vi "Edgertronic-:get_current_settings copy.vi"(4 "GET Command":string="/get_current_settings", 5 "Setup":T1={"URL"="130.64.16.195", "remote port"=80, "mode (standard)"=enum."Standard"}) -> (0 "error out":errorcluster, 1 "Current Settings:":T2={"Connection Information:"="", "Requested Genlock "="20140911165611", "Min Frame Clocks "="20140911165611", "Is Seq Clk Freq "="20140911165611", "Pretrigger Frames "="20140911165611", "Duration "="20140911165611", "Overclock "="20140911165611", "Requested Horizontal "="20140911165611", "Frames "="20140911165611", "Requested Pretrigger "="20140911165611", "Words per Frame "="20140911165611", "Buffer End "="20140911165611", "Clocks per Frame  "="20140911165611", "Requested Duration "="20140911165611", "Pretrigger "="20140911165611", "Post-trigger Frames "="20140911165611", "Vertical "="20140911165611", "Requested Vertical "="20140911165611", "Reqested Frame Rate "="20140911165611", "Frame Rate "="20140911165611", "Horizontal "="20140911165611", "Clocks per Exposure "="20140911165611", "Digital Gain "="20140911165611", "Exposure "="20140911165611", "Genlock "="20140911165611", "Analog Gain "="20140911165611", "Subsample "="20140911165611", "Requested Exposure "="20140911165611", "Iso "="20140911165611", "Requested Overclock "="20140911165611", "Requested Subsample "="20140911165611", "Requested Iso"="20140911165611", "FPGA Temp"="20140911165611", "Posttrigger Duration"="20140911165611", "dacvrefadc"="20140911165611", "Is Temp"="20140911165611", "Pretrigger Duration"="20140911165611"}, 2 "Data Out from Camera":string="HTTP/1.0 200 OK\r\nContent-Type: text/html; charset=utf-8\r\nContent-Length: 313\r\nConnection: close\r\nDate: Tue, 16 Jun 2015 13:54:12 GMT\r\nServer: lighttpd/1.4.11 (edgertonic slow motion camera)\r\n\r\n{\"build_date\": \"20150112\", \"sw_build_date\": \"20140911165611\", \"fpga_initialized\": 1, \"hardware_revision\": 6, \"model_number\": 1, \"home_dir\": \"/home/root/ss-web\", \"ir_filter\": 1, \"mac_addr\": \"00:1B:C5:09:61:4D\", \"serial_console_enabled\": false, \"serial_number\": 333, \"fpga_version\": 70, \"hardware_configuration\": 1}")   [LabVIEW 2012]
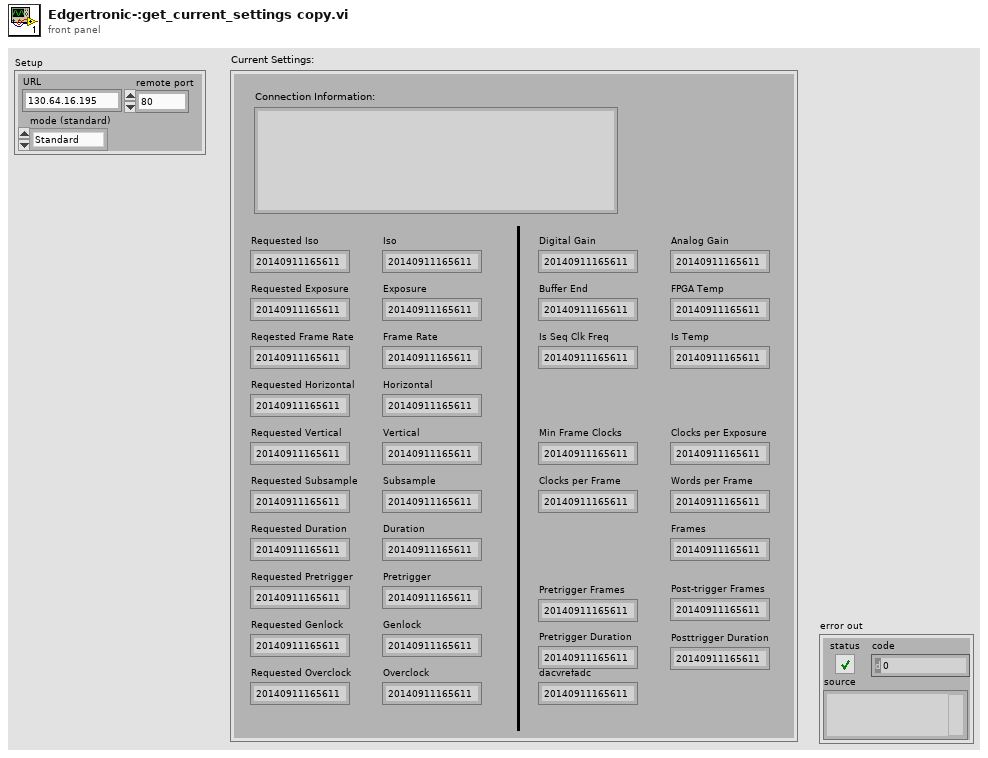
[diagram p1: front panel]
types:
  T1 = cluster{"URL":string, "remote port":u16, "mode (standard)":enum16{"Standard", "Buffered", "CRLF", "Immediate"}}
  T2 = cluster{"Connection Information:":string, "Requested Genlock ":string, "Min Frame Clocks ":string, "Is Seq Clk Freq ":string, "Pretrigger Frames ":string, "Duration ":string, "Overclock ":string, "Requested Horizontal ":string, "Frames ":string, "Requested Pretrigger ":string, "Words per Frame ":string, "Buffer End ":string, "Clocks per Frame  ":string, "Requested Duration ":string, "Pretrigger ":string, "Post-trigger Frames ":string, "Vertical ":string, "Requested Vertical ":string, "Reqested Frame Rate ":string, "Frame Rate ":string, "Horizontal ":string, "Clocks per Exposure ":string, "Digital Gain ":string, "Exposure ":string, "Genlock ":string, "Analog Gain ":string, "Subsample ":string, "Requested Exposure ":string, "Iso ":string, "Requested Overclock ":string, "Requested Subsample ":string, "Requested Iso":string, "FPGA Temp":string, "Posttrigger Duration":string, "dacvrefadc":string, "Is Temp":string, "Pretrigger Duration":string}
  T3 = cluster{"Parameter":string, "Parameter 2":string, "Parameter 3":string, "Parameter 4":string, "Parameter 5":string, "Parameter 6":string, "Parameter 7":string, "Parameter 8":string, "Parameter 9":string, "Parameter 10":string, "Parameter 11":string, "Parameter 12":string, "Parameter 13":string, "Parameter 14":string, "Parameter 15":string, "Parameter 16":string, "Parameter 17":string, "Parameter 18":string, "Parameter 19":string, "Parameter 20":string, "Parameter 21":string, "Parameter 22":string, "Parameter 23":string, "Parameter 24":string, "Parameter 25":string, "Parameter 26":string, "Parameter 27":string, "Parameter 28":string, "Parameter 29":string, "Parameter 30":string, "Parameter 31":string, "Parameter 32":string, "Parameter 33":string, "Parameter 34":string, "Parameter 35":string, "Parameter 36":string}
  T4 = cluster{"[0]":string, "[1]":string, "[2]":string, "[3]":string, "[4]":string, "[5]":string, "[6]":string, "[7]":string, "[8]":string, "[9]":string, "[10]":string, "[11]":string, "[12]":string, "[13]":string, "[14]":string, "[15]":string, "[16]":string, "[17]":string, "[18]":string, "[19]":string, "[20]":string, "[21]":string, "[22]":string, "[23]":string, "[24]":string, "[25]":string, "[26]":string, "[27]":string, "[28]":string, "[29]":string, "[30]":string, "[31]":string, "[32]":string, "[33]":string, "[34]":string, "[35]":string}
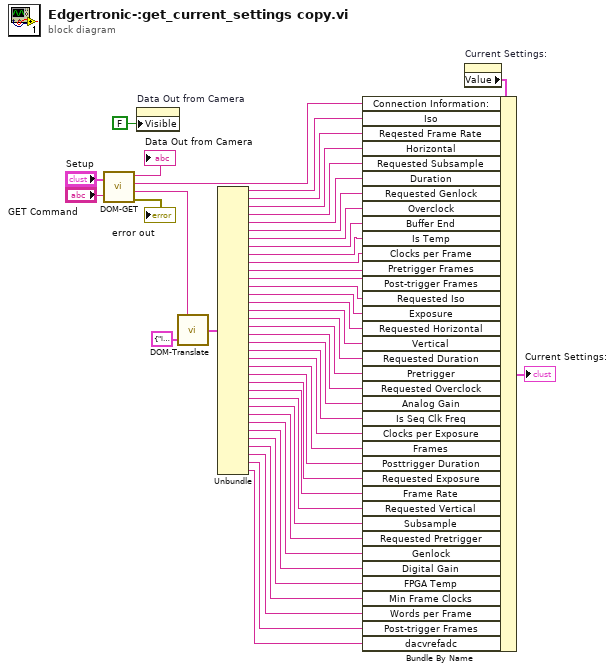
[diagram p0: block diagram]
diagram:
  n1 = call <userlib>:"DOM-GET.vi"("Setup"="Setup", "GET Command"="GET Command") -> ("Data Out from Camera"=→"Data Out from Camera":string, "Connection Information"=w2:string, "Value String"=w1:string, "error out"=→"error out":errorcluster)
  n2 = property on="Data Out from Camera" class="Str"("Visible"=FALSE) -> ()  [unwired: 2 in, 2 out]
  n3 = call <userlib>:"DOM-Translate.vi"("Parameter Cluster in"=T3 {"Parameter"="iso", "Parameter 2"="requested_frame_rate", "Parameter 3"="horizontal", "Parameter 4"="requested_subsample", "Parameter 5"="duration", "Parameter 6"="requested_genlock", "Parameter 7"="overclock", "Parameter 8"="buffer_end", "Parameter 9"="is_temp", "Parameter 10"="clocks_per_frame", "Parameter 11"="pretrigger_frames", "Parameter 12"="post_trigger_duration", "Parameter 13"="requested_iso", "Parameter 14"="exposure", "Parameter 15"="requested_horizontal", "Parameter 16"="vertical", "Parameter 17"="requested_duration", "Parameter 18"="pretrigger", "Parameter 19"="requested_overclock", "Parameter 20"="analog_gain", "Parameter 21"="is_seq_clk_freq", "Parameter 22"="clocks_per_exposure", "Parameter 23"="frames", "Parameter 24"="pre_trigger_duration", "Parameter 25"="requested_exposure", "Parameter 26"="frame_rate", "Parameter 27"="requested_vertical", "Parameter 28"="subsample", "Parameter 29"="requested_pretrigger", "Parameter 30"="genlock", "Parameter 31"="digital_gain", "Parameter 32"="fpga_temp", "Parameter 33"="min_frame_clocks", "Parameter 34"="words_per_frame", "Parameter 35"="posttrigger_frames", "Parameter 36"="dacvrefadc"}, "Value Data in"=w1) -> ("Value Cluster out"=w46:T4)
  n4 = Unbundle(w46) -> ("[0]"=w45:string, "[1]"=w44:string, "[2]"=w43:string, "[3]"=w42:string, "[4]"=w41:string, "[5]"=w40:string, "[6]"=w39:string, "[7]"=w38:string, "[8]"=w37:string, "[9]"=w36:string, "[10]"=w35:string, "[11]"=w34:string, "[12]"=w33:string, "[13]"=w32:string, "[14]"=w31:string, "[15]"=w30:string, "[16]"=w29:string, "[17]"=w28:string, "[18]"=w27:string, "[19]"=w26:string, "[20]"=w25:string, "[21]"=w24:string, "[22]"=w23:string, "[23]"=w22:string, "[24]"=w21:string, "[25]"=w20:string, "[26]"=w19:string, "[27]"=w18:string, "[28]"=w17:string, "[29]"=w16:string, "[30]"=w15:string, "[31]"=w14:string, "[32]"=w13:string, "[33]"=w12:string, "[34]"=w11:string, "[35]"=w10:string)
  n5 = property on="Current Settings:" class="Clust (strict)"() -> ("Value"=w9:T2)  [unwired: 2 in, 2 out]
  n6 = Bundle By Name(cluster=w9, "Connection Information:"=w2, "Iso"=w45, "Reqested Frame Rate"=w44, "Horizontal"=w43, "Requested Subsample"=w42, "Duration"=w41, "Requested Genlock"=w40, "Overclock"=w39, "Buffer End"=w38, "Is Temp"=w37, "Clocks per Frame"=w36, "Pretrigger Frames"=w35, "Post-trigger Frames"=w34, "Requested Iso"=w33, "Exposure"=w32, "Requested Horizontal"=w31, "Vertical"=w30, "Requested Duration"=w29, "Pretrigger"=w28, "Requested Overclock"=w27, "Analog Gain"=w26, "Is Seq Clk Freq"=w25, "Clocks per Exposure"=w24, "Frames"=w23, "Posttrigger Duration"=w22, "Requested Exposure"=w21, "Frame Rate"=w20, "Requested Vertical"=w19, "Subsample"=w18, "Requested Pretrigger"=w17, "Genlock"=w16, "Digital Gain"=w15, "FPGA Temp"=w14, "Min Frame Clocks"=w13, "Words per Frame"=w12, "Post-trigger Frames"=w11, "dacvrefadc"=w10) -> (→"Current Settings:":T2)
